vi "Init.vi"(8 "error in (no error)":errorcluster, 11 "VI in":refnum<vi>) -> (0 "error out":errorcluster)   [LabVIEW 2019, in "TemplateModule.lvlib"]
uses:
  TemplateModule.lvlib
  Tools/Tools.lvlib
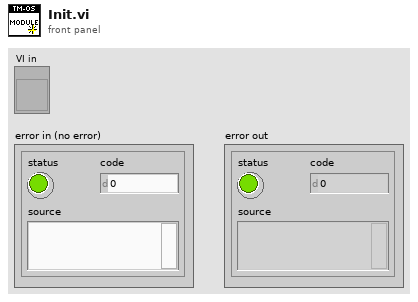
[diagram p1: front panel]
types:
  T1 = enum32{"Bad", "Idle", "Run top level", "Running"}
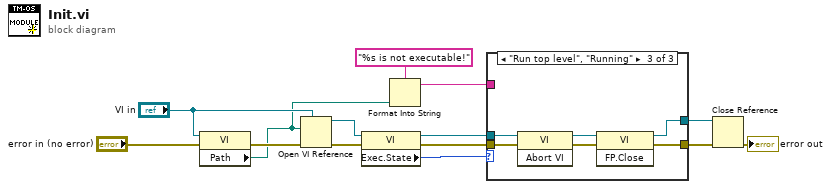
[diagram p0: block diagram]
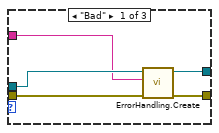
[diagram p2: hidden frame]
diagram:
  n1 = property class="VI"(reference="VI in", error in="error in (no error)") -> (error out=w12:errorcluster, "Path"=w2:path)  [unwired: 1 out]
  n2 = Open VI Reference(type specifier VI Refnum (for type only)="VI in", vi path=w2, error in (no error)=w12) -> (vi reference=w1:refnum<vi>, error out=w13:errorcluster)  [unwired: 3 in]
  n3 = property class="VI"(reference=w1, error in=w13) -> (reference out=w4:refnum<vi>, error out=w6:errorcluster, "Exec.State"=w3:T1)
  n4 = Format Into String(format string="%s is not executable!" ("explanation"), w2) -> (resulting string=w10:string)  [unwired: 2 in, 1 out]
  n5 = case shown="\"Run top level\", \"Running\"" w3 {
    tunnel: [w17 w20 w21] -> w7
    tunnel: w6 -> [w18 w20 w26]
    tunnel: [w16 w19 w22] -> w5
    tunnel: w4 -> [w16 w19 w25]
    tunnel: w10 -> [w15 _ _]
    frame "Bad" {
      n6 = call "ErrorHandling.Create.vi"("error in"=w18, "explanation"=w15) -> ("error out"=w17:errorcluster)  [unwired: 9 in]
    }
    frame "Idle" {
    }
    frame "Run top level", "Running" {
      n7 = invoke class="VI" method="Abort VI"(reference=w25, error in=w26) -> (reference out=w23:refnum<vi>, error out=w24:errorcluster)  [unwired: 1 in, 1 out]
      n8 = invoke class="VI" method="FP.Close"(reference=w23, error in=w24) -> (reference out=w22:refnum<vi>, error out=w21:errorcluster)  [unwired: 1 in, 1 out]
    }
  }
  n9 = Close Reference(reference=w5, error in (no error)=w7) -> (error out=→"error out":errorcluster)
